vi "SIM Bicycle.vi"(6 "initial condition":dbl[](array[numeric])=[0.0, 0.0, 0.0], 7 "handbrake":dbl=1.0, 9 "L":dbl=1.0, 10 "gamma":dbl, 11 "v":dbl) -> (1 "theta":dbl, 2 "y":dbl, 3 "x":dbl)   [LabVIEW 2017]
uses:
  <vilib>/Simulation/Implementation/Shared/SIMSCR Execution Mode.ctl
  <vilib>/Simulation/Scripting/Companion Diagram/SimConfigNode/SimParams.ctl
  <vilib>/Simulation/Scripting/Companion Diagram/SimConfigNode/_simSolvers.ctl
  <vilib>/Platform/TimedLoop/XDataNode/timing_clust.ctl
  <vilib>/Platform/TimedLoop/XDataNode/nitl_modes.ctl
  <vilib>/Platform/TimedLoop/XDataNode/wakeup.ctl
  <vilib>/Simulation/Param Hierarchy/Typedefs/SIMPH Param Control Actions.ctl
  <vilib>/Simulation/Implementation/Shared/SIM limit type.ctl
  <vilib>/Simulation/Implementation/Shared/NILVSim_ParamChanged.vi
  <vilib>/Simulation/Implementation/Shared/NILVSim_FinishedLate.vi
  <vilib>/Simulation/Implementation/Shared/NILVSIM_BeginStep.vi
  <vilib>/Simulation/Nonlinear/Implementation/NILVSim Saturation.llb/SIM Saturation (scalar).vi
  <vilib>/Simulation/Nonlinear/Implementation/NILVSim RateLimiter.llb/SIM RateLimiter (scalar).vi
  <vilib>/Simulation/ContinuousLinear/Implementation/NILVSim Integrator new.llb/SIM Integrator Distributor (vector).vi
  <vilib>/Simulation/ContinuousLinear/Implementation/NILVSim Integrator new.llb/SIM Integrator Collector (vector).vi
  <vilib>/Simulation/Implementation/Shared/NILVSim_Manager.vi
  <vilib>/Utility/error.llb/Clear Errors.vi
  <vilib>/Simulation/Implementation/Shared/NILVSim_FinalizeModel.vi
  <vilib>/Simulation/Implementation/Shared/SIM Unbundle Sim Info.vi
  <vilib>/Simulation/Implementation/Shared/SIMSH Read Queue.vi
  <vilib>/Simulation/Implementation/Shared/NILVSim_Initialize.vi
  <vilib>/Simulation/Utility/Implementation/NILVSim Get Time and IsAcceptedStep.vi
  <vilib>/Simulation/Implementation/Shared/NILVSim_GetModelError.vi
  <vilib>/Simulation/Implementation/Shared/SIM SimErrorHandler.vi
  <vilib>/Simulation/Implementation/Shared/SIM Bundle Sim Info.vi
  <vilib>/Simulation/Scripting/Companion Diagram/SimConfigNode/SimDog.xnode
  <vilib>/Platform/TimedLoop/XDataNode/XDataNode.xnode
  <vilib>/Simulation/Implementation/XNodeFramework/SimXNode/SimX.xnode
  <vilib>/Simulation/ContinuousLinear/Implementation/NILVSim Integrator new.llb/SIM Integrator (vector).vi
  <vilib>/Platform/TimedLoop/XDataNode/XDNodeRunTimeDep.lvlib
  <vilib>/Simulation/Implementation/Shared/NI_SIM_Implementation.lvlib
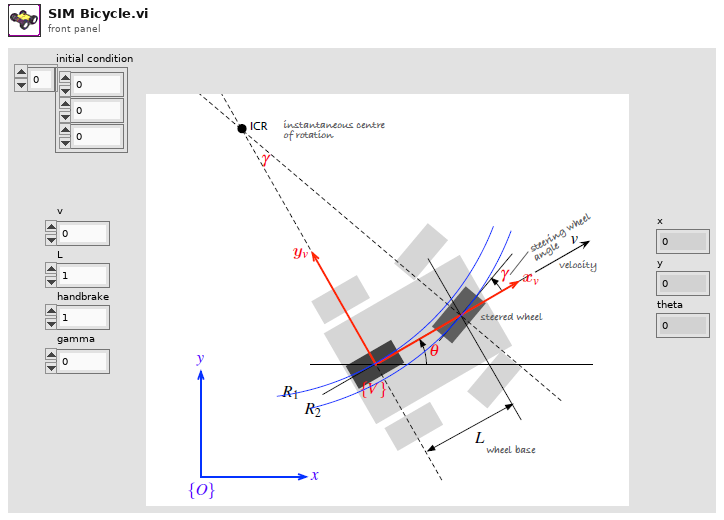
[diagram p1: front panel]
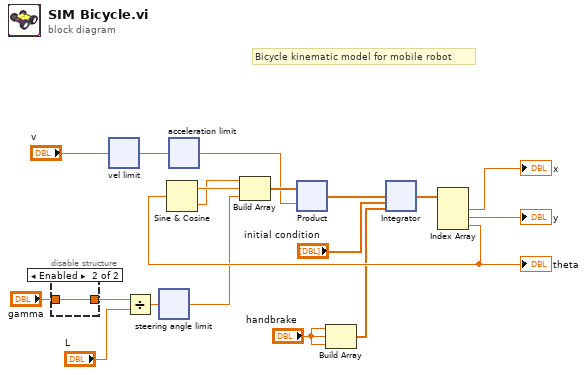
[diagram p0: block diagram]
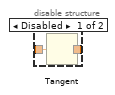
[diagram p2: hidden frame]
diagram:
  # "Bicycle kinematic model for mobile robot"
  n1 = disable-structure "Diagram Disable Structure" shown="Enabled" {
    disable-tunnel: [w21 w22] -> w9
    disable-tunnel: "gamma" -> [w20 w22]
    frame Disabled {
      n2 = Tangent(1:w20) -> (0:w21:dbl)
    }
    frame Enabled {
    }
  }
  n3 = xnode "vel limit"("input"="v") -> ("output"=w19:dbl)  [unwired: 4 in]
  n4 = Divide ("Divide 2")(x=w9, y="L") -> (x/y=w6:dbl)
  n5 = xnode "steering angle limit"("input"=w6) -> ("output"=w5:dbl)  [unwired: 4 in]
  n6 = xnode "acceleration limit"("input"=w19) -> ("output"=w10:dbl)  [unwired: 4 in]
  n7 = Build Array ("Build Array 2")("handbrake", "handbrake", "handbrake") -> (w1:dbl[])
  n8 = Sine & Cosine(0:w12) -> (1:w4:dbl, 2:w3:dbl)
  n9 = Build Array(w3, w4, w5) -> (w18:dbl[])
  n10 = xnode "Product"("Operand1"=w18, "Operand2"=w10) -> ("Result"=w16:dbl[])
  n11 = xnode "Integrator"("input"=w16, "initial condition"="initial condition", "reset"=w1) -> ("output"=w15:dbl[])  [unwired: 7 in, 2 out]
  n12 = Index Array ("Index Array 4")(array=w15) -> (element #1=→"x":dbl, element #2=→"y":dbl, element #3=w12:dbl)  [unwired: 3 in]
  "theta" <- w12
